vi "Talon Test 2016.vi"() -> ()   [LabVIEW 2015]
doc: "This example shows how to control motor speed using CAN Jaguar and a quadrature encoder. For details setting up and understanding CAN Jaguar, see the Can Jaguar Fundamentals tutorial accessable from the LabVIEW Getting Started Window.\n\nTo control the motor speed, a PID control loop runs on the Jaguar. Notice that the encoder is wired directly to the Jaguar. One advantage of this is that the PID control does not use resources on the roboRIO. One disadvantage is that the PID code cannot be viewed or changed. However, the control can be tuned by changing the PID Parameters.\n\nOn the diagram, notice that the PID tuning parameters are only applied once before the motor is enabled. To learn about changing PID parameters while the program is running, see the CAN Position Control Encoder example. Since the control loop runs on the Jaguar, the LabVIEW loop delay is set to a slow 100ms. In fact the only reason this loop needs to run is to send a new set speed and read the actual speed.\n\nCorrect tuning parameters for a PID controller are dependent on the complete system of the motor and the load. It will be difficult to tune this system if there is no load attached to the motor. While this example is not a PID tutorial, the following information may help in understanding how to tune your PID control system.\n\nP (proportional) depends on the present error, I (integral) on the accumulation of past errors, and D (derivative) is a prediction of future errors, based on the current rate of change. The proportional parameter (P) will reduce the rise time and will reduce, but never eliminate, the steady-state error. The integral parameter (I) will eliminate the steady-state error, but may make the transient response worse. The derivative parameter (D) will increase the stability of the system, reducing the overshoot, and improving the transient response. The effects of each parameter are summarized in a table on the front panel.\n\nThis example expects a USB cable connected from your development PC to the Type B USB Jack (next to the power input) on the roboRIO.\n\nThis example requires the Driver Station to be running with Teleoperated Enabled."
uses:
  <vilib>/Rock Robotics/WPI/CAN/TalonSRX/WPI_CANTalonSRX_APIFeedbackSelect.ctl
  <vilib>/Rock Robotics/WPI/CAN/TalonSRX/WPI_CANTalonSRX_APIControlMode.ctl
  <vilib>/Rock Robotics/WPI/MotorControl/WPI_MotorControlOpenCANTalonSRX.vi
panel:
  in  "I Zone":dbl=0.01
  in  "Switches Normally Open":bool
  in  "Reverse Limit Switch":bool
  in  "Forward Limit Switch":bool
  in  "stop":bool
  in  "Tab Control":T1(tab)
  out "Voltage Feedback Chart":cluster{dbl, dbl}(graph)
  out "Speed Feedback Chart":cluster{dbl, dbl}(graph)
  out "Position Feedback Chart":cluster{dbl, dbl}(graph)
  out "Potentiometer Position Feedback":cluster{dbl, dbl}(graph)
  in  "Motor Address":u64
  in  "Combo Box":string(combo)
  out "Error Out":errorcluster
  in  "Error In":errorcluster
  out "Test Running":string
  out "A/D Value":dbl
  out "Percent VBus":dbl
  out "Actual Position (Rotations)":dbl
  in  "Target Value":dbl
  in  "I":dbl
  in  "F":dbl=0.01
  in  "D":dbl
  in  "P":dbl=1.0
  out "Actual Speed (RPM)":dbl
  # "Set these inputs before running."
  # "Tuning parameters"
  # "Feed-Forward"
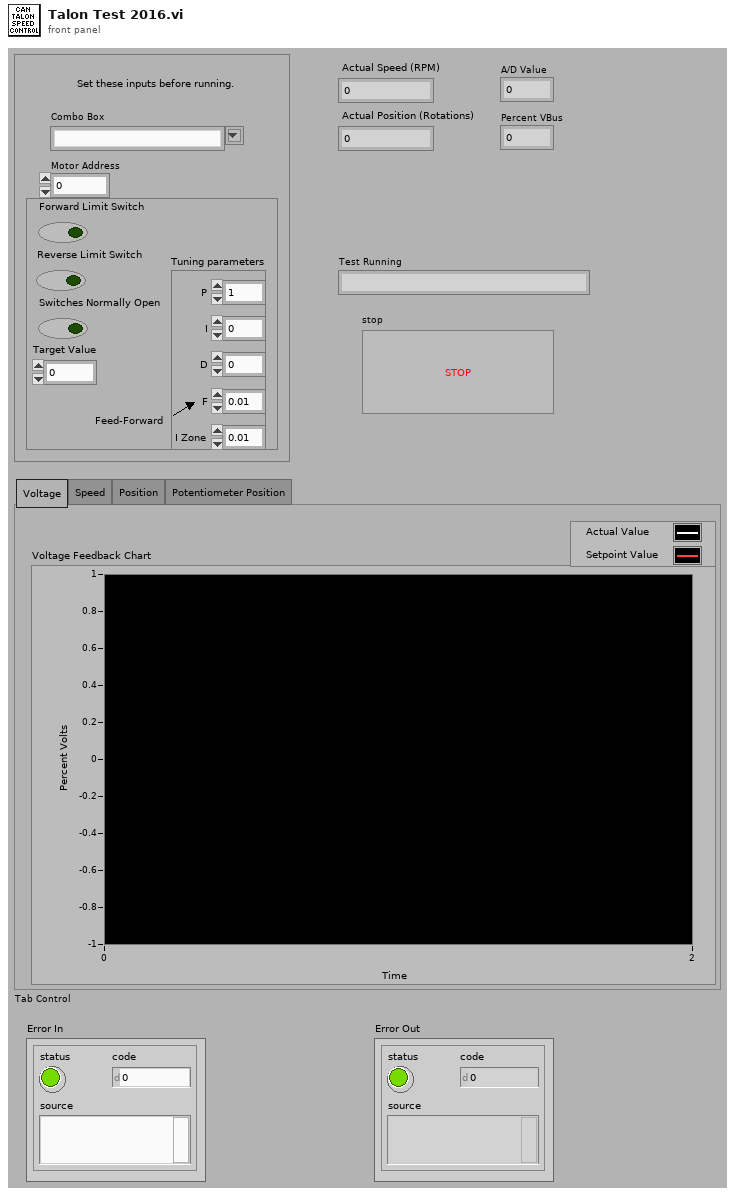
[diagram p1: front panel]
types:
  T1 = enum32{"Voltage", "Speed", "Position", "Potentiometer Position"}
  T2 = typedef "WPI_CANTalonSRX_APIFeedbackSelect.ctl" = enum16{"Digital Quadrature Encoder", "Analog Potentiometer", "Analog Encoder", "Count on Quad-A (Rising-Edge)", "Count on Quad-A (Falling-Edge)", "CTR Magnetic Enc (Absolute)", "CTR Magnetic Enc (Relative)", "Pulse Width"}
  T3 = typedef "WPI_CANTalonSRX_APIControlMode.ctl" = enum8{"Percent VBus", "Speed", "Position", "Slave", "Unchanged / Invalid", "Voltage Compensation", "Current", "Motion Profile"}
  T4 = typedef "WPI_MotorControlDeviceRef.ctl" = cluster{"DeviceStatus":errorcluster, "Type":T5, "PWM":cluster{"PWM Channel":T6, "DeadBand":T7}, "CAN":cluster{"Device Number":u8, "Control Mode":T8, "Semaphore":T9, "Max Vout":dbl, "TalonSRX Control Mode":T3}, "Invert":bool}
  T5 = typedef "WPI_MotorControlType.ctl" = enum16{"PWM", "CAN", "CANTalonSRX"}
  T6 = typedef "FPGA_DIOPWMChannel.ctl" = enum8{"PWM 0", "PWM 1", "PWM 2", "PWM 3", "PWM 4", "PWM 5", "PWM 6", "PWM 7", "PWM 8", "PWM 9", "PWM MXP 0", "PWM MXP 1", "PWM MXP 2", "PWM MXP 3", "PWM MXP 4", "PWM MXP 5", "PWM MXP 6", "PWM MXP 7", "PWM MXP 8", "PWM MXP 9", "Invalid"}
  T7 = typedef "WPI_PWMDeadband.ctl" = cluster{"Name":string, "maxPositivePwm":i32, "minPositivePwm":i32, "centerPwm":i32, "maxNegativePwm":i32, "minNegativePwm":i32, "angularRange":u16}
  T8 = typedef "WPI_CANJaguar_ControlMode.ctl" = enum8{"Percent VBus", "Current", "Speed", "Position", "Voltage"}
  T9 = typedef "Semaphore RefNum" = refnum<k1>
  T10 = typedef "WPI_CANTalonSRX_GlobalStatus.ctl" = cluster{"Applied Throttle":dbl, "Module Enabled":bool, "CAN Error":errorcluster, "Closed Loop Error":dbl, "Forward Limit Switch Closed":bool, "Reverse Limit Switch Closed":bool, "Sensor Position":dbl, "Sensor Velocity":dbl, "Current":dbl, "Sticky Fault - Over Temp":bool, "Sticky Fault - Under Voltage":bool, "Sticky Fault - Forward Limit":bool, "Sticky Fault - Reverse Limit":bool, "Sticky Fault - Forward Soft Limit":bool, "Sticky Fault - Reverse Soft Limit":bool, "Brake is Enabled":bool, "Encoder Position":dbl, "Encoder Velocity":dbl, "Encoder Index Count":dbl, "Encoder A Pin State":bool, "Encoder B Pin State":bool, "Encoder Index Pin State":bool, "Analog In":dbl, "Analog In Velocity":dbl, "Temperature (C)":dbl, "Battery Voltage":dbl, "Control 5 Is Supported":bool, "Current Profile Slot Select":dbl, "Pos Div 8":bool, "Vel Div 4":bool, "Pulse Width Position":i32, "Pulse Width Velocity":i32, "Pulse Width Rise To Rise (us)":i32, "Pulse Width Rise To Fall (us)":i32, "Mot Prof Active Is Under Run":bool, "Mot Prof Active Has Under Run":bool, "Mot Prof Active Is Last":bool, "Mot Prof Active Velocity Only":bool, "Mot Prof Active Is Valid":bool, "Mot Prof Buffer Is Full":bool, "Mot Prof Active Profile Slot Select":i32, "Mot Prof NextID":i32, "Mot Prof Count":i32, "Mot Prof Active Velocity":dbl, "Mot Prof Active Position":dbl, "Mot Prof Output Enable":i32}
  T11 = cluster{"Applied Throttle":dbl, "Target Value":dbl}
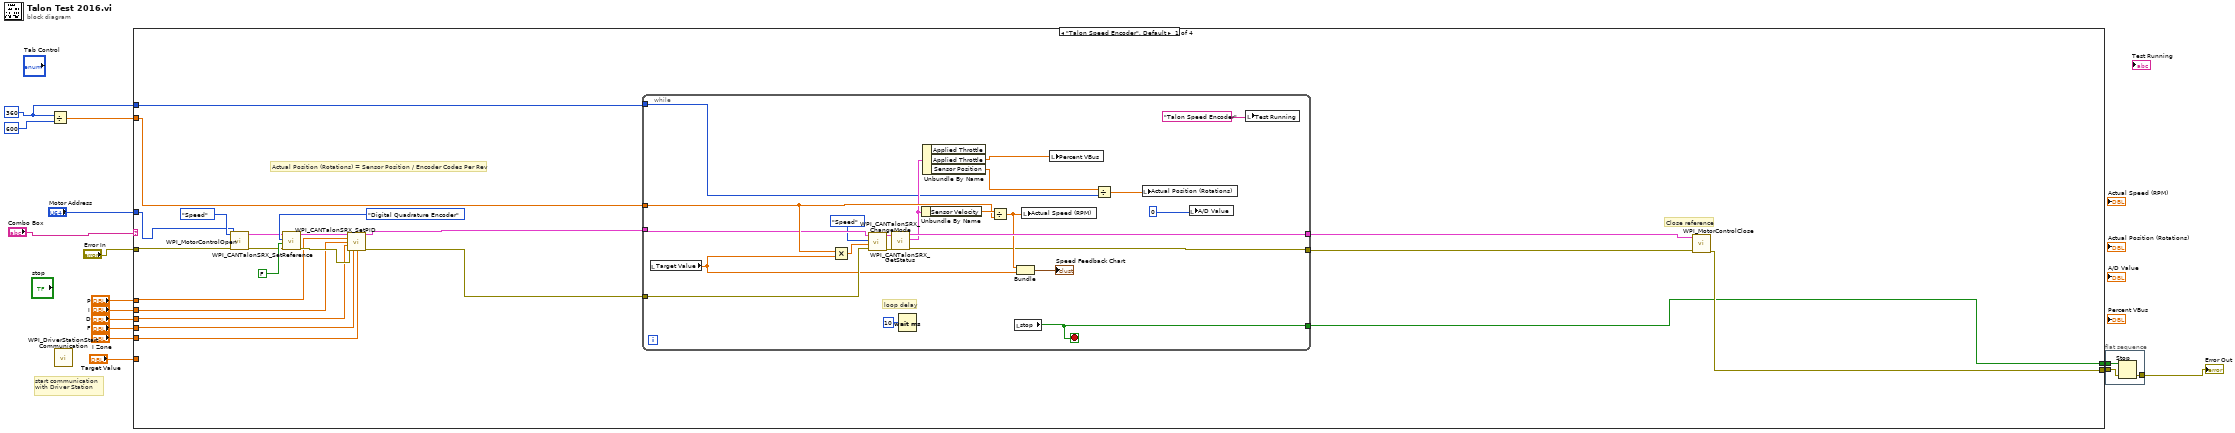
[diagram p0: block diagram]
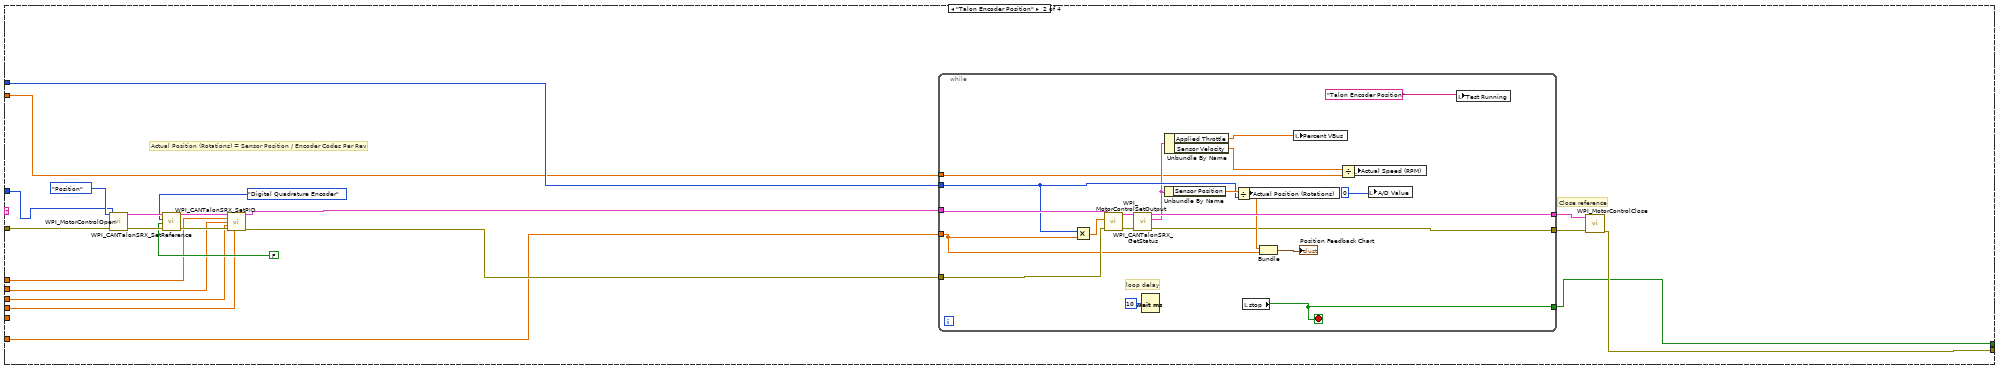
[diagram p2: hidden frame]
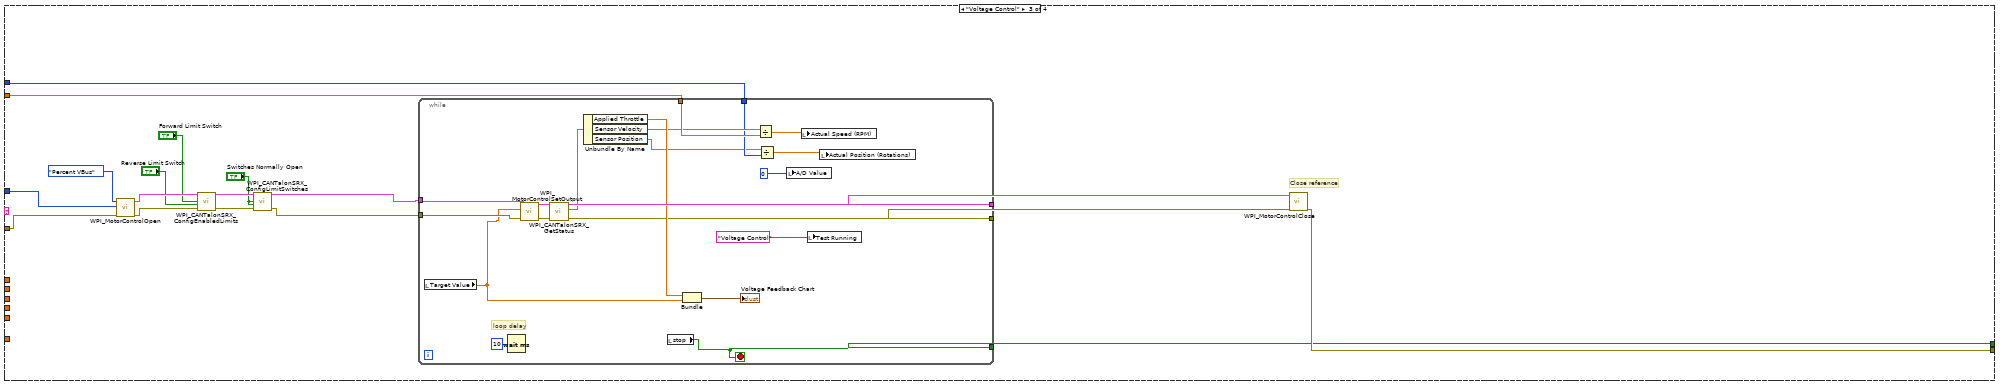
[diagram p3: hidden frame]
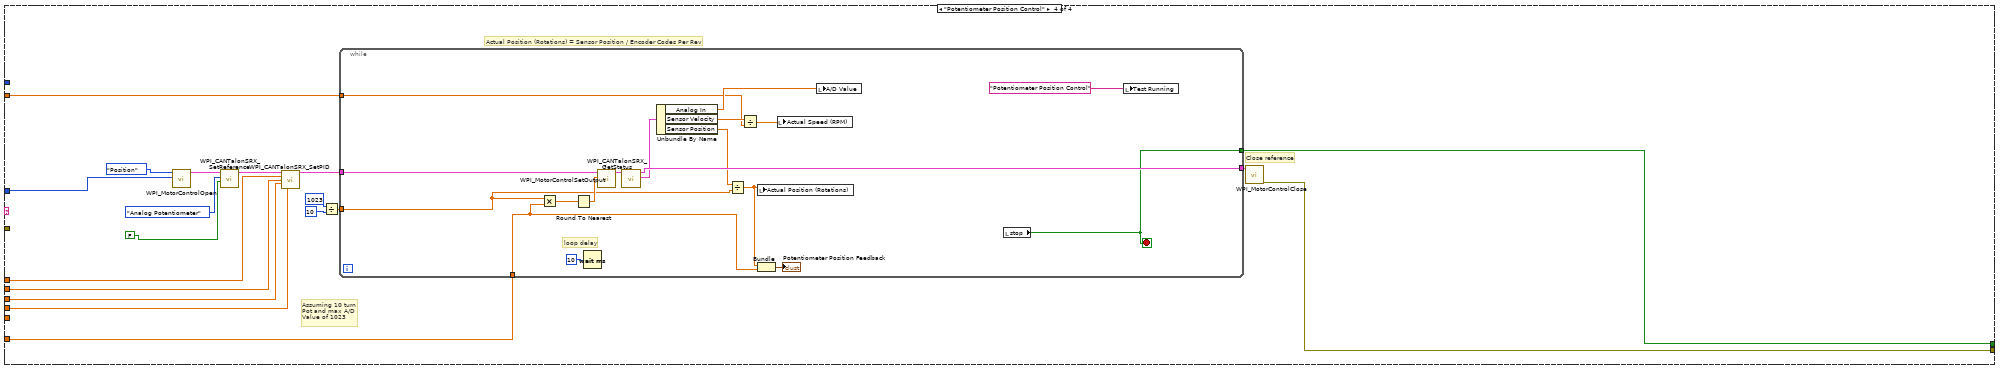
[diagram p4: hidden frame]
diagram:
  w13 = 360
  # "start communication with Driver Station"
  n1 = Divide(x=w13, y=600) -> (x/y=w14:dbl)
  n2 = call <vilib>:"WPI_DriverStationStart Communication.vi"() -> ()  [unwired: 2 in, 10 out]
  n3 = case shown="\"Talon Speed Encoder\", Default" "Combo Box" {
    tunnel: w14 -> [w25 w60 w116 w142]
    tunnel: w13 -> [w26 w61 w117 _]
    tunnel: "Error In" -> [w23 w69 w114 _]
    tunnel: [w18 w63 w113 w143] -> w3
    tunnel: "P" -> [w22 w68 _ w148]
    tunnel: "I" -> [w21 w67 _ w147]
    tunnel: "D" -> [w20 w66 _ w141]
    tunnel: "F" -> [w19 w65 _ w146]
    tunnel: "Target Value" -> [_ w64 _ w145]
    tunnel: "Motor Address" -> [w24 w70 w115 w149]
    tunnel: [w17 w62 w112 w144] -> w4
    tunnel: "I Zone" -> [w16 _ _ _]
    frame "Talon Speed Encoder", Default {
      # "Actual Position (Rotations) = Sensor Position / Encoder Codes Per Rev"
      # "Close reference"
      n4 = call-poly <vilib>:"WPI_MotorControlOpen.vi"("error in (no error)"=w23, "Device Number"=w24, "Control Mode"=WPI_CANTalonSRX_APIControlMode."Speed") -> ("error out"=w30:errorcluster, "MotorControlDeviceRef"=w33:T4)  [unwired: 2 in, 5 out]
      n5 = call <vilib>:"WPI_CANTalonSRX_SetReference.vi"("error in (no error)"=w30, "Reverse Feedback Sensor"=FALSE, "Feedback Reference"=WPI_CANTalonSRX_APIFeedbackSelect."Digital Quadrature Encoder", "CAN Talon SRX Ref"=w33) -> ("error out"=w29:errorcluster, "CAN Talon SRX Ref"=w32:T4)  [unwired: 6 in]
      n6 = call <vilib>:"WPI_CANTalonSRX_SetPID.vi"("CAN Talon SRX Ref"=w32, "P"=w22, "I"=w21, "D"=w20, "error in (no error)"=w29, "F"=w19, "I Zone"=w16) -> ("CAN Talon SRX Ref"=w31:T4, "error out"=w28:errorcluster)  [unwired: 7 in]
      n7 = while {
        tunnel: [w46] -> w17
        tunnel: w31 -> [w44]
        tunnel: [w58] -> w37
        tunnel: w25 -> [w55]
        tunnel: w26 -> [w49]
        tunnel: w28 -> [w43]
        tunnel: [w47] -> w27
        stop <- w46 stop-if-true
        # "loop delay"
        n8 = local read "Target Value"() -> (w38:dbl)
        n9 = Multiply(x=w55, y=w38) -> (x*y=w40:dbl)
        n10 = call <vilib>:"WPI_CANTalonSRX_ChangeMode.vi"("error in (no error)"=w43, "Output"=w40, "Control Mode"=WPI_CANTalonSRX_APIControlMode."Speed", "CAN Talon SRX Ref"=w44) -> ("error out"=w42:errorcluster, "CAN Talon SRX Ref"=w41:T4)  [unwired: 6 in]
        n11 = call <vilib>:"WPI_CANTalonSRX_GetStatus.vi"("error in (no error)"=w42, "CAN Talon SRX Ref"=w41) -> ("error out"=w47:errorcluster, "Talon SRX Status"=w51:T10, "CAN Talon SRX Ref"=w58:T4)  [unwired: 7 in]
        n12 = Wait (ms)(milliseconds to wait=u32 10) -> ()  [unwired: 1 out]
        n13 = Unbundle By Name(w51) -> ("Sensor Velocity"=w57:dbl)
        n14 = Unbundle By Name(w51) -> ("Applied Throttle"=w50:dbl, "Sensor Position"=w48:dbl)  [unwired: 1 out]
        n15 = Divide(x=w57, y=w55) -> (x/y=w54:dbl)
        n16 = local read "stop"() -> (w46:bool)
        n17 = Bundle(w54, "Target Value"=w38) -> (→"Speed Feedback Chart":cluster{dbl, "Target Value":dbl})  [unwired: 1 in]
        n18 = local write "Actual Speed (RPM)"(w54) -> ()
        n19 = local write "Percent VBus"(w50) -> ()
        n20 = Divide(x=w48, y=w49) -> (x/y=w53:dbl)
        n21 = local write "Actual Position (Rotations)"(w53) -> ()
        n22 = local write "A/D Value"(0) -> ()
        n23 = local write "Test Running"("Talon Speed Encoder") -> ()
      }
      n24 = call <vilib>:"WPI_MotorControlClose.vi"("error in (no error)"=w27, "MotorControlDevRef"=w37) -> ("error out"=w18:errorcluster)  [unwired: 9 in]
    }
    frame "Talon Encoder Position" {
      # "Actual Position (Rotations) = Sensor Position / Encoder Codes Per Rev"
      # "Close reference"
      n25 = call-poly <vilib>:"WPI_MotorControlOpen.vi"("error in (no error)"=w69, "Device Number"=w70, "Control Mode"=WPI_CANTalonSRX_APIControlMode."Position") -> ("error out"=w78:errorcluster, "MotorControlDeviceRef"=w75:T4)  [unwired: 2 in, 5 out]
      n26 = call <vilib>:"WPI_CANTalonSRX_SetReference.vi"("error in (no error)"=w78, "Reverse Feedback Sensor"=FALSE, "Feedback Reference"=WPI_CANTalonSRX_APIFeedbackSelect."Digital Quadrature Encoder", "CAN Talon SRX Ref"=w75) -> ("error out"=w79:errorcluster, "CAN Talon SRX Ref"=w76:T4)  [unwired: 6 in]
      n27 = call <vilib>:"WPI_CANTalonSRX_SetPID.vi"("CAN Talon SRX Ref"=w76, "P"=w68, "I"=w67, "D"=w66, "error in (no error)"=w79, "F"=w65) -> ("CAN Talon SRX Ref"=w77:T4, "error out"=w80:errorcluster)  [unwired: 8 in]
      n28 = while {
        tunnel: [w83] -> w62
        tunnel: w77 -> [w96]
        tunnel: [w101] -> w71
        tunnel: w61 -> [w95]
        tunnel: w80 -> [w89]
        tunnel: [w87] -> w81
        tunnel: w64 -> [w86]
        tunnel: w60 -> [w85]
        stop <- w83 stop-if-true
        # "loop delay"
        n29 = Multiply(x=w95, y=w86) -> (x*y=w98:dbl)
        n30 = call <vilib>:"WPI_MotorControlSetOutput.vi"("error in (no error)"=w89, "Output"=w98, "MotorControlDevRef"=w96) -> ("error out"=w88:errorcluster, "MotorControlDevRef"=w100:T4)  [unwired: 6 in, 1 out]
        n31 = call <vilib>:"WPI_CANTalonSRX_GetStatus.vi"("error in (no error)"=w88, "CAN Talon SRX Ref"=w100) -> ("error out"=w87:errorcluster, "Talon SRX Status"=w91:T10, "CAN Talon SRX Ref"=w101:T4)  [unwired: 7 in]
        n32 = Wait (ms)(milliseconds to wait=u32 10) -> ()  [unwired: 1 out]
        n33 = Unbundle By Name(w91) -> ("Sensor Position"=w99:dbl)
        n34 = Unbundle By Name(w91) -> ("Applied Throttle"=w84:dbl, "Sensor Velocity"=w90:dbl)
        n35 = Divide(x=w99, y=w95) -> (x/y=w94:dbl)
        n36 = local read "stop"() -> (w83:bool)
        n37 = local write "Actual Position (Rotations)"(w94) -> ()
        n38 = Bundle(w94, "Target Value"=w86) -> (→"Position Feedback Chart":cluster{dbl, "Target Value":dbl})  [unwired: 1 in]
        n39 = local write "Percent VBus"(w84) -> ()
        n40 = Divide(x=w90, y=w85) -> (x/y=w93:dbl)
        n41 = local write "Actual Speed (RPM)"(w93) -> ()
        n42 = local write "A/D Value"(0) -> ()
        n43 = local write "Test Running"("Talon Encoder Position") -> ()
      }
      n44 = call <vilib>:"WPI_MotorControlClose.vi"("error in (no error)"=w81, "MotorControlDevRef"=w71) -> ("error out"=w63:errorcluster)  [unwired: 9 in]
    }
    frame "Voltage Control" {
      # "Close reference"
      n45 = call-poly <vilib>:"WPI_MotorControlOpen.vi"("error in (no error)"=w114, "Device Number"=w115, "Control Mode"=WPI_CANTalonSRX_APIControlMode."Percent VBus") -> ("error out"=w108:errorcluster, "MotorControlDeviceRef"=w111:T4)  [unwired: 2 in, 5 out]
      n46 = call <vilib>:"WPI_CANTalonSRX_ConfigEnabledLimits.vi"("CAN Talon SRX Ref"=w111, "Forward Limit Switch Enable"="Forward Limit Switch", "Reverse Limit Switch Enable"="Reverse Limit Switch", "error in (no error)"=w108) -> ("CAN Talon SRX Ref"=w110:T4, "error out"=w107:errorcluster)  [unwired: 10 in]
      n47 = call <vilib>:"WPI_CANTalonSRX_ConfigLimitSwitches.vi"("CAN Talon SRX Ref"=w110, "Forward Limit Switch Normally Open"="Switches Normally Open", "Reverse Limit Switch Normally Open"="Switches Normally Open", "error in (no error)"=w107) -> ("CAN Talon SRX Ref"=w109:T4, "error out"=w106:errorcluster)  [unwired: 10 in]
      n48 = while {
        tunnel: [w123] -> w112
        tunnel: w109 -> [w136]
        tunnel: [w139] -> w119
        tunnel: w116 -> [w135]
        tunnel: w117 -> [w131]
        tunnel: w106 -> [w127]
        tunnel: [w125] -> w118
        stop <- w123 stop-if-true
        # "loop delay"
        n49 = local read "Target Value"() -> (w121:dbl)
        n50 = Wait (ms)(milliseconds to wait=u32 10) -> ()  [unwired: 1 out]
        n51 = call <vilib>:"WPI_MotorControlSetOutput.vi"("error in (no error)"=w127, "Output"=w121, "MotorControlDevRef"=w136) -> ("error out"=w126:errorcluster, "MotorControlDevRef"=w138:T4)  [unwired: 6 in, 1 out]
        n52 = call <vilib>:"WPI_CANTalonSRX_GetStatus.vi"("error in (no error)"=w126, "CAN Talon SRX Ref"=w138) -> ("error out"=w125:errorcluster, "Talon SRX Status"=w137:T10, "CAN Talon SRX Ref"=w139:T4)  [unwired: 7 in]
        n53 = Unbundle By Name(w137) -> ("Applied Throttle"=w134:dbl, "Sensor Velocity"=w132:dbl, "Sensor Position"=w130:dbl)
        n54 = local read "stop"() -> (w123:bool)
        n55 = Bundle("Applied Throttle"=w134, "Target Value"=w121) -> (→"Voltage Feedback Chart":T11)  [unwired: 1 in]
        n56 = Divide(x=w132, y=w135) -> (x/y=w133:dbl)
        n57 = Divide(x=w130, y=w131) -> (x/y=w129:dbl)
        n58 = local write "A/D Value"(0) -> ()
        n59 = local write "Actual Speed (RPM)"(w133) -> ()
        n60 = local write "Test Running"("Voltage Control") -> ()
        n61 = local write "Actual Position (Rotations)"(w129) -> ()
      }
      n62 = call <vilib>:"WPI_MotorControlClose.vi"("error in (no error)"=w118, "MotorControlDevRef"=w119) -> ("error out"=w113:errorcluster)  [unwired: 9 in]
    }
    frame "Potentiometer Position Control" {
      # "Assuming 10 turn\nPot and max A/D\nValue of 1023"
      # "Actual Position (Rotations) = Sensor Position / Encoder Codes Per Rev"
      # "Close reference"
      n63 = call-poly <vilib>:"WPI_MotorControlOpen.vi"("Device Number"=w149, "Control Mode"=WPI_CANTalonSRX_APIControlMode."Position") -> ("MotorControlDeviceRef"=w156:T4)  [unwired: 3 in, 6 out]
      n64 = call <vilib>:"WPI_CANTalonSRX_SetReference.vi"("Reverse Feedback Sensor"=FALSE, "Feedback Reference"=WPI_CANTalonSRX_APIFeedbackSelect."Analog Potentiometer", "CAN Talon SRX Ref"=w156) -> ("CAN Talon SRX Ref"=w155:T4)  [unwired: 7 in, 1 out]
      n65 = call <vilib>:"WPI_CANTalonSRX_SetPID.vi"("CAN Talon SRX Ref"=w155, "P"=w148, "I"=w147, "D"=w141, "F"=w146) -> ("CAN Talon SRX Ref"=w152:T4)  [unwired: 9 in, 1 out]
      n66 = Divide(x=1023, y=10) -> (x/y=w153:dbl)
      n67 = while {
        tunnel: [w161] -> w144
        tunnel: w152 -> [w171]
        tunnel: [w176] -> w159
        tunnel: w153 -> [w165]
        tunnel: w145 -> [w168]
        tunnel: w142 -> [w163]
        stop <- w161 stop-if-true
        # "loop delay"
        n68 = Multiply(x=w165, y=w168) -> (x*y=w170:dbl)
        n69 = Round To Nearest(number=w170) -> (nearest integer value=w169:dbl)
        n70 = Wait (ms)(milliseconds to wait=u32 10) -> ()  [unwired: 1 out]
        n71 = call <vilib>:"WPI_MotorControlSetOutput.vi"("Output"=w169, "MotorControlDevRef"=w171) -> ("MotorControlDevRef"=w175:T4)  [unwired: 7 in, 2 out]
        n72 = call <vilib>:"WPI_CANTalonSRX_GetStatus.vi"("CAN Talon SRX Ref"=w175) -> ("Talon SRX Status"=w174:T10, "CAN Talon SRX Ref"=w176:T4)  [unwired: 8 in, 1 out]
        n73 = Unbundle By Name(w174) -> ("Analog In"=w167:dbl, "Sensor Velocity"=w164:dbl, "Sensor Position"=w173:dbl)
        n74 = Divide(x=w173, y=w165) -> (x/y=w162:dbl)
        n75 = Divide(x=w164, y=w163) -> (x/y=w166:dbl)
        n76 = local write "Actual Position (Rotations)"(w162) -> ()
        n77 = Bundle(w162, "Target Value"=w168) -> (→"Potentiometer Position Feedback":cluster{dbl, "Target Value":dbl})  [unwired: 1 in]
        n78 = local write "Actual Speed (RPM)"(w166) -> ()
        n79 = local write "A/D Value"(w167) -> ()
        n80 = local read "stop"() -> (w161:bool)
        n81 = local write "Test Running"("Potentiometer Position Control") -> ()
      }
      n82 = call <vilib>:"WPI_MotorControlClose.vi"("MotorControlDevRef"=w159) -> ("error out"=w143:errorcluster)  [unwired: 10 in]
    }
  }
  n83 = flat-sequence {
    tunnel: w4 -> [w179]
    tunnel: w3 -> [w178]
    tunnel: [w178] -> w2
    frame #0 {
      n84 = Stop(stop? (T)=w179) -> ()
    }
  }
  "Error Out" <- w2
